vi "_OLS_Main_Rev4.vi"() -> ()   [LabVIEW 2024]
uses:
  Control Definitions/Def_PumpSpeed.ctl
  Control Definitions/Def TestState.ctl
  Control Definitions/DEF_PumpCtlRefs.ctl
  Control Definitions/DEF_Results.ctl
  Control Definitions/DEF_ Results3.ctl
  Control Definitions/Def_ATPStatus.ctl
  Control Definitions/DEF_TestInfo.ctl
  Control Definitions/Registry Keys.ctl
  Control Definitions/Global 2.vi
  Control Definitions/Global 1.vi
panel:
  out "Report Path":path
  out "Pefump VISA Ref":refnum<visa-resource-name>
  out "Test Info":T1={"Job Number"="", "Unit Number"="", "Serial Number"="", "Technician Name"="", "Calibration Date"="Cal Date", "Calibrator"="Cal by", "Calibration Slope"="M", "Calibration Offset"="B", "Config File Name"="Cal Date"}
  out "Results":T2 {"Resistor 2" format="%.1f"; "Drain" format="%.3f"; "Resistor" format="%.1f"; "Fill" format="%.3f"}
  in  "End Prog":bool=TRUE
  out "Test Index Out":i32
  out "PumpCtlRef out":T5
  out "TEST State Out":T6
  in  "Pump Speed":T7
  out "Ch B  Sim":dbl=101.0
  out "Ch A  Sim":dbl=200.0
  out "Root Path":path=path "C:/AllenProjects/PWC-OLS"
  out "Time(ms)":dbl=1249.4499999994114
  in  "ChA":dbl(slide)=24.489795918367346 scale=0.0..1200.0
  in  "ChB":dbl(slide)=36.73469387755102 scale=0.0..1200.0
  in  "ChB +100":bool
  in  "ChA +100":bool
  in  "Check":bool
  in  "DUT":i16=1
  in  "Pump JOG":bool=TRUE
  in  "Run Test":bool
  out "Pump \nStatus":bool=TRUE
  out "DataQ\nStatus":bool=TRUE
  in  "Level SP":dbl(slide)=8.0 scale=8.5..2.0
  in  "Level PV":dbl(slide)=7.715118932422306 scale=8.5..2.0
  out "Level":dbl=7.715118932422306 format="%.3f"
  in  "Drain":bool
  in  "Fill":bool
  in  "Simulate":bool
  out "TEST Name":string="OLR001--cal"
  out "DataQ Input":T8(graph)={"ChA Ohms"=100.83065830421491, "ChB Ohms"=100.0340857774357, "Laser (raw)"=1.9040000438690186}
  out "Time Stamp":timestamp=timestamp(3810639016.2712703 s since 1904-01-01)
  in  "stop":bool
  out "ChB Ohms":dbl=100.0340857774357 format="%.1f"
  out "ChA Ohms":dbl=100.79497115454612 format="%.1f"
  # "Calibration & Scaling Table\n               Tank         Key          Ref\n               Scale        Level        Measure\nEmpty\n\n\nFull"
  # "8.0      1.7752      7.844\n\n2.6      6.112        3.511"
  # "CHA             Resistance     Fill     Resistance   Drain"
  # "CHB           Resistance     Fill     Resistance   Drain"
  # "PUMP"
  # "Simulated Resistor In"
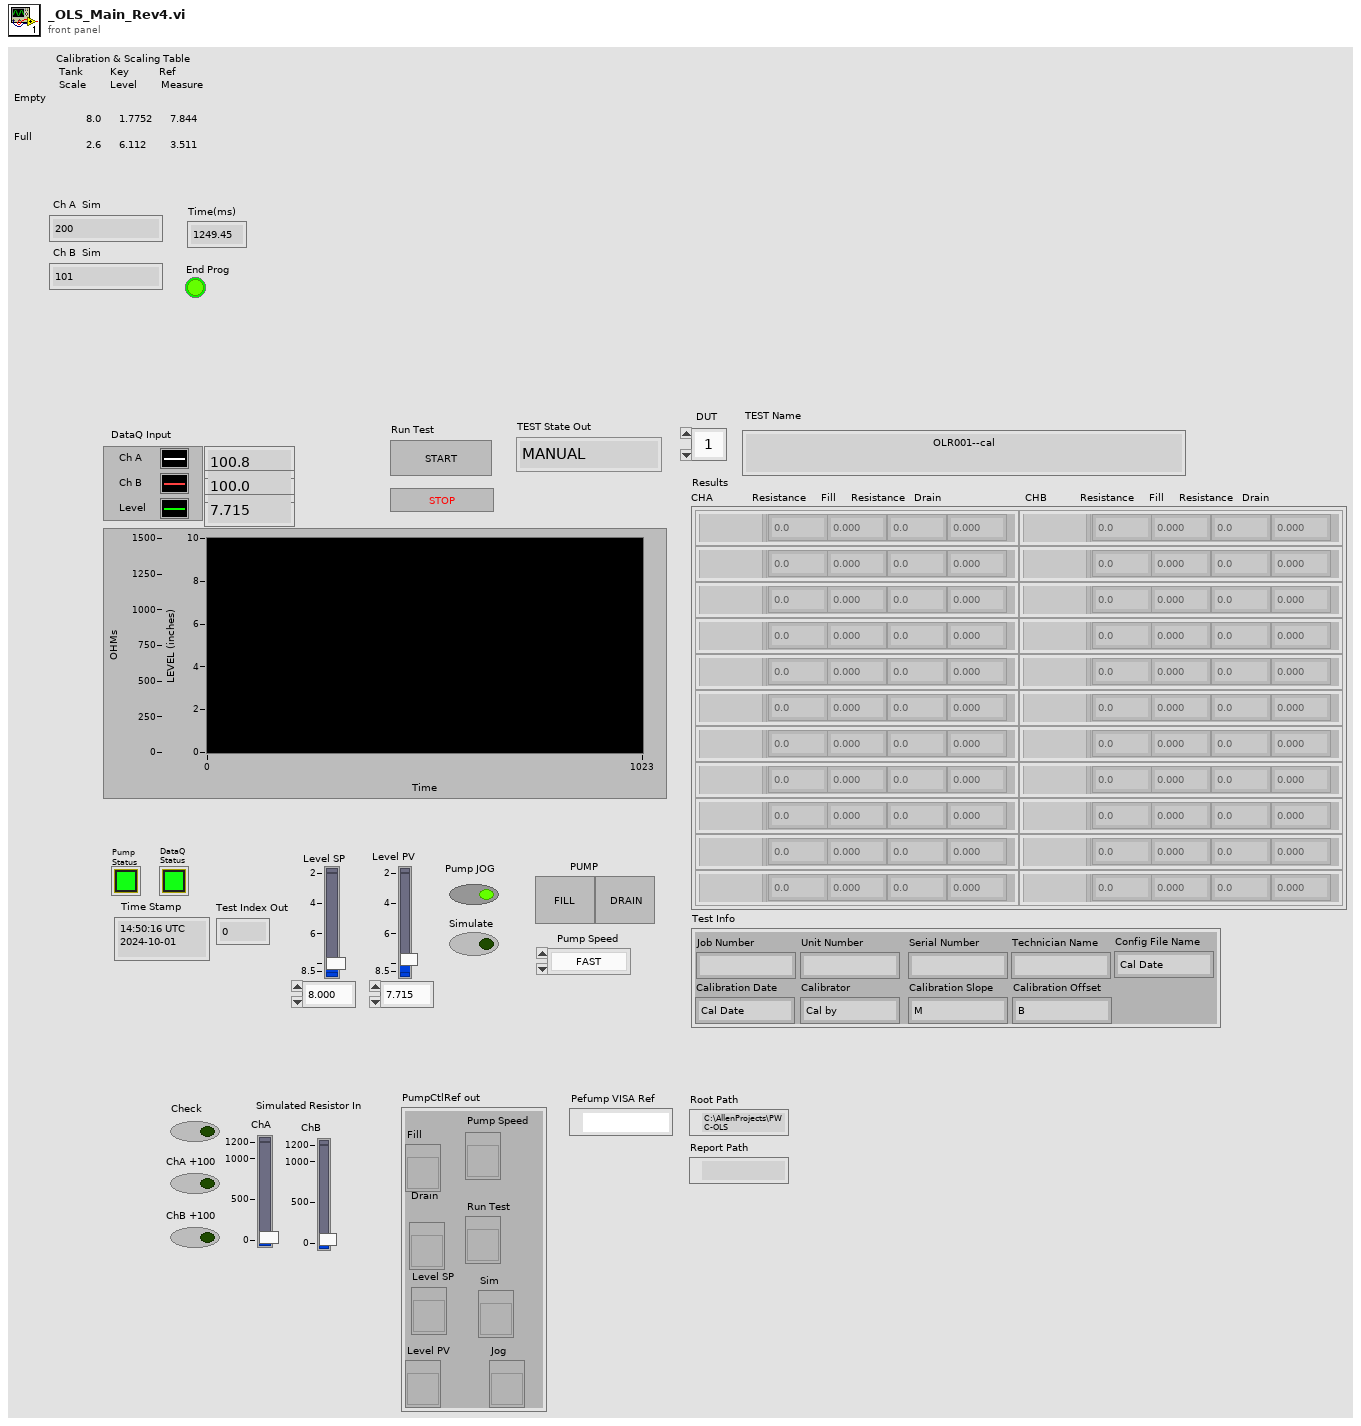
[diagram p1: front panel]
types:
  T1 = typedef "DEF_TestInfo.ctl" = cluster{"Job Number":string, "Unit Number":string, "Serial Number":string, "Technician Name":string, "Calibration Date":string, "Calibrator":string, "Calibration Slope":string, "Calibration Offset":string, "Config File Name":string}
  T2 = typedef "DEF_Results.ctl" = T3[][]
  T3 = typedef "DEF_ Results3.ctl" = cluster{"Fill":dbl, "Status":T4, "Resistor":dbl, "Drain":dbl, "Resistor 2":dbl}
  T4 = typedef "Def_ATPStatus.ctl" = i16
  T5 = typedef "DEF_PumpCtlRefs.ctl" = cluster{"Fill ":refnum<vi>, "Drain":refnum<vi>, "Level PV":refnum<vi>, "Pump Speed":refnum<vi>, "Run Test":refnum<vi>, "Sim":refnum<vi>, "Jog":refnum<vi>, "Level SP":refnum<vi>}
  T6 = typedef "Def TestState.ctl" = enum16{"MANUAL", "Start", "Pre-Fill", "Pre-Fill Measure", "Pre-Drain", "Pre-Drain Measure", "Init-Record", "Load Fill Spec", "Filling Hi", "Wait1", "Record Fill", "Load Drain Spec", "Draining Lo", "Wait2", "Record Drain", "Empty", "Done"}
  T7 = typedef "Def_PumpSpeed.ctl" = enum16{"FAST", "SLOW", "CREEP", "STOP"}
  T8 = cluster{"ChA Ohms":dbl, "ChB Ohms":dbl, "Laser (raw)":dbl}
  T9 = typedef "Registry Keys.ctl" = enum16{"Report Files Key", "Config Files Key"}
  T10 = cluster{"Pump \nStatus":refnum<vi>, "DataQ\nStatus":refnum<vi>}
  T11 = typedef "DEF_FullConfig.ctl" = cluster{"Bench Params":T12, "Test Params":dbl[][], "Pump Params":T13, "DataQ Params":T14, "Pump Control Ref":T5, "Bench Status":T15}
  T12 = typedef "DEF_BenchParams.ctl" = cluster{"Relative Root Name":string, "Values":cluster{"Step Levels":dbl, "Resistor Tolerence":dbl, "Sample Rate":dbl, "Resistor":dbl, "Wait Time":dbl}, "Report Template path":path, "Test Type":string, "Config File Name":string, "Config 2 Use":string, "Skip Pre Lube":bool}
  T13 = typedef "DEF_PumpParams.ctl" = cluster{"Empty Inches":dbl, "Full Inches":dbl, "RNG_SLOW":dbl, "RNG_CREEP":dbl, "RNG_STOP ":dbl, "VISA resource name":refnum<visa-resource-name>, "SPD_SLOW":i32, "SPD_CREEP":i32, "SPD_FAST":i32, "Zero template":path, "zero  Settle sec":i32, "Laser Slope":sgl, "Laser Offset":sgl, "Sim Fill Rate":sgl, "Cal Date":string, "Cal Technician":string}
  T14 = typedef "DEF_DataqParams.ctl" = cluster{"Visa Name":string, "Num Chan":i32, "Cal Coef":cluster{"M":dbl, "B":dbl}[], "Scale ":i32, "Cal Date":string, "Cal Technicain":string}
  T15 = typedef "DEF_BenchStatus.ctl" = cluster{"Pump Status":refnum<vi>, "Instrumnet\n Status":refnum<vi>}
  T16 = enum16{"MANUAL", "Start", "Filling", "FULL", "Draining", "EMPTY", "Done"}
  T17 = typedef "DEF_LevelOut.ctl" = cluster{"Laser ":cluster{"Raw":sgl, "Scaled":dbl}, "Level PV":dbl, "Fill":bool, "Drain":bool}
  T18 = typedef "DEF_SpecsOut.ctl" = cluster{"aSpecsTable":T19[], "Pump CtlRef In":T5, "TEST State Out":T6, "TEST Index":i32, "Drain!Fill":bool}
  T19 = typedef "Def Spec RNG.ctl" = cluster{"Specs":dbl[], "LUT Status":T20}
  T20 = typedef "Ded LUT_Status.ctl" = cluster{"ChA/!ChB":bool, "Drain/!Fill":bool, "In Range?":bool, "Switch Range?":bool, "Measure R?":bool, "Vaild R?":bool, "Index(n)":i32, "Index(n)-1":i32, "Index Max":i32, "Index(n-1)":i32}
  T21 = typedef "Def Measure.ctl" = cluster{"ChA R":dbl, "ChB R":dbl, "Level PV":dbl}
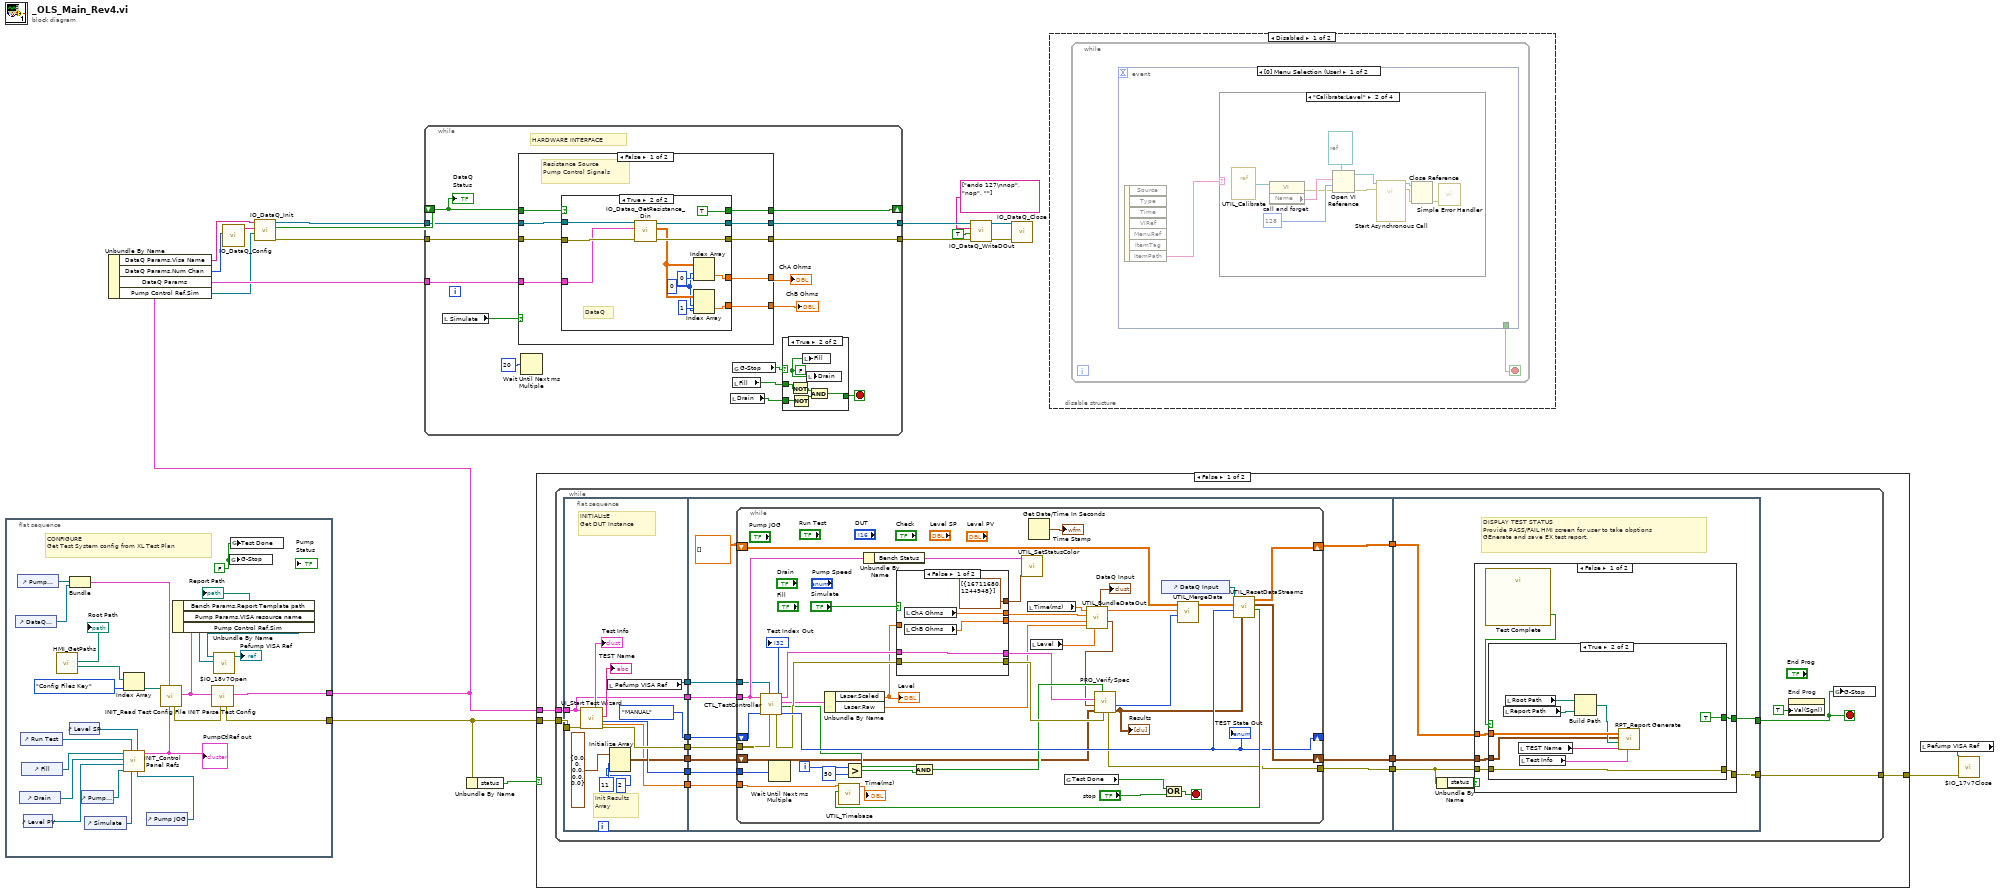
[diagram p0: block diagram]
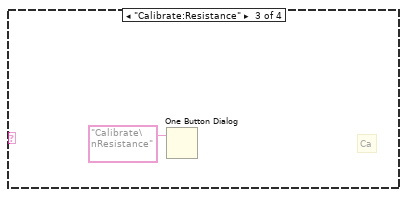
[diagram p3: hidden frame]
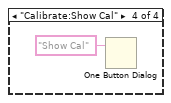
[diagram p4: hidden frame]
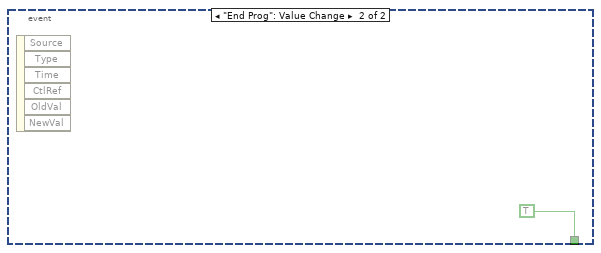
[diagram p5: hidden frame]
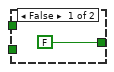
[diagram p7: hidden frame]
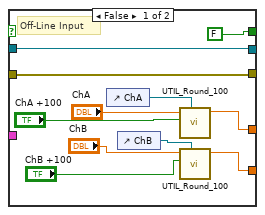
[diagram p8: hidden frame]
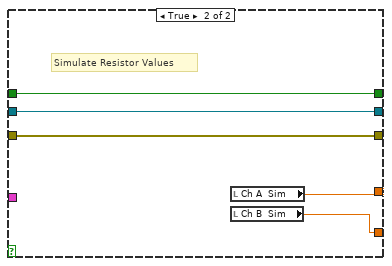
[diagram p9: hidden frame]
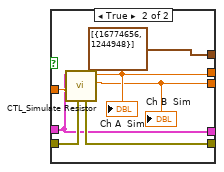
[diagram p10: hidden frame]
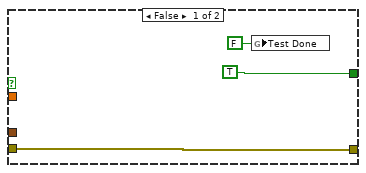
[diagram p11: hidden frame]
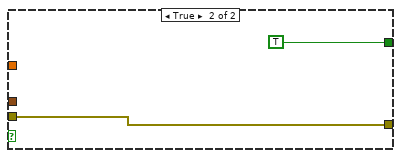
[diagram p12: hidden frame]
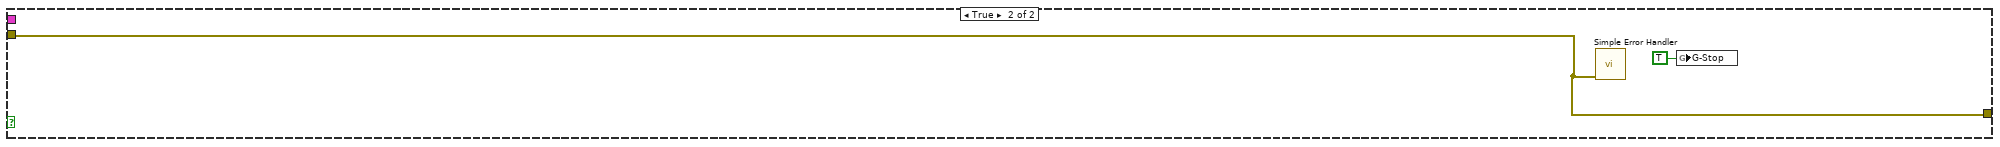
[diagram p13: hidden frame]
diagram:
  n1 = flat-sequence {
    tunnel: [w25] -> w18
    tunnel: [w39] -> w17
    frame #0 {
      w34 = FALSE ("G-Stop")
      # "CONFIGURE\nGet Test System config from XL Test Plan"
      n2 = control-ref of="DataQ\nStatus"() -> (w36:refnum<vi>)
      n3 = control-ref of="Pump \nStatus"() -> (w43:refnum<vi>)
      n4 = control-ref of="Drain"() -> (w44:refnum<vi>)
      n5 = control-ref of="Run Test"() -> (w40:refnum<vi>)
      n6 = control-ref of="Fill"() -> (w41:refnum<vi>)
      n7 = control-ref of="Level PV"() -> (w42:refnum<vi>)
      n8 = call "HMI_GetPaths.vi"() -> ("Default Paths"=w30:path[], "Root Path"=→"Root Path":path)  [unwired: 10 in]
      n9 = Bundle("Pump \nStatus"=w43, "DataQ\nStatus"=w36) -> (w28:T10)  [unwired: 1 in]
      n10 = control-ref of="Level SP"() -> (w35:refnum<vi>)
      n11 = control-ref of="Pump Speed"() -> (w32:refnum<vi>)
      n12 = control-ref of="Simulate"() -> (w38:refnum<vi>)
      n13 = Index Array(array=w30, index=Registry_Keys."Config Files Key" ("Reg Key")) -> (element=w29:path)
      n14 = control-ref of="Pump JOG"() -> (w37:refnum<vi>)
      n15 = call "INIT_Control Panel Refs.vi"("Jog"=w37, "Level SP"=w35, "Sim"=w38, "Run Test"=w40, "Pump Speed"=w32, "Level PV"=w42, "Drain"=w44, "Fill"=w41) -> ("PumpCtlRef out"=w27:T5)  [unwired: 3 in]
      "PumpCtlRef out" <- w27
      n16 = call "INIT_Read Test Config File.vi"("Pump Control Ref"=w27, "Bench Status"=w28, "Path"=w29) -> ("FullConfig"=w24:T11, "error out"=w26:errorcluster)  [unwired: 7 in]
      n17 = Unbundle By Name(w24) -> ("Bench Params.Report Template path"=→"Report Path":path, "Pump Params.VISA resource name"=w23:refnum<visa-resource-name>, "Pump Control Ref.Sim"=w20:refnum<vi>)
      n18 = call "INIT Parse Test Config.vi"("error in"=w26, "Full Config In"=w24) -> ("Full Config Out"=w39:T11, "error out"=w25:errorcluster)  [unwired: 8 in]
      n19 = call "$IO_18v7Open.vi"("Pump Control Ref.Sim"=w20, "Runtime VISA name"=w23) -> ("VISA Refnum out"=→"Pefump VISA Ref":refnum<visa-resource-name>)  [unwired: 8 in, 1 out]
      n20 = global write "Global 1.vi" "G-Stop"(w34) -> ()
      n21 = global write "Global 2.vi" "Test Done"(w34) -> ()
    }
  }
  n22 = Unbundle By Name(w17) -> ("DataQ Params.Visa Name"=w5:string, "DataQ Params.Num Chan"=w6:i32, "DataQ Params"=w4:T14, "Pump Control Ref.Sim"=w1:refnum<vi>)
  n23 = call "IO_DataQ_Config.vi"("Num Chan"=w6) -> ("Init Message"=w16:string[])  [unwired: 10 in]
  n24 = call "IO_DataQ_Init.vi"("Pump Control Ref.Sim"=w1, "Command\nList"=w16, "RunTime VISA name"=w5) -> ("error out"=w14:errorcluster, "Connected?"=w13:bool, "VISA resource name out"=w15:refnum<visa-resource-name>)  [unwired: 6 in]
  n25 = while {
    tunnel: w15 -> [w57]
    tunnel: w14 -> [w56]
    tunnel: [w54] -> w12
    tunnel: [w55] -> w10
    shift-right: [w53] -> _
    shift-left: w13 -> [w52]
    tunnel: w4 -> [w45]
    stop <- w49 stop-if-true
    # "HARDWARE INTERFACE"
    n26 = local read "Simulate"() -> (w51:bool)
    n27 = case shown="False" w51 {
      tunnel: [w75 w100] -> w58
      tunnel: [w74 w99] -> w46
      tunnel: w57 -> [w68 w102]
      tunnel: w56 -> [w69 w101]
      tunnel: [w73 w101] -> w55
      tunnel: [w72 w102] -> w54
      tunnel: [w71 w103] -> w53
      tunnel: w52 -> [w70 w103]
      tunnel: w45 -> [w67 _]
      frame False {
        # "Resistance Source\nPump Control Signals"
        n28 = case shown="True" w70 {
          tunnel: [w79 w95] -> w75
          tunnel: [w80 w92] -> w74
          tunnel: [w81 w98] -> w72
          tunnel: [w82 w97] -> w73
          tunnel: [FALSE TRUE] -> w71
          tunnel: w69 -> [w82 w88]
          tunnel: w68 -> [w81 w89]
          tunnel: w67 -> [_ w87]
          frame False {
            # "Off-Line Input"
            n29 = control-ref of="ChA"() -> (w78:refnum<vi>)
            n30 = control-ref of="ChB"() -> (w76:refnum<vi>)
            n31 = call "UTIL_Round_100.vi"("Num Refnum"=w78, "100"="ChA +100", "IN"="ChA") -> ("OUT"=w80:dbl)  [unwired: 8 in]
            n32 = call "UTIL_Round_100.vi"("Num Refnum"=w76, "100"="ChB +100", "IN"="ChB") -> ("OUT"=w79:dbl)  [unwired: 8 in]
          }
          frame True {
            w91 = 0 ("disabled index (col)")
            # "DataQ"
            n33 = call "IO_Dataq_GetResistance_Din.vi"("error in (no error)"=w88, "Dataq Params"=w87, "VISA Refnum in"=w89) -> ("error out"=w97:errorcluster, "Analog"=w93:dbl[][], "VISA Refnum out"=w98:refnum<visa-resource-name>)  [unwired: 5 in, 1 out]
            n34 = Index Array(array=w93, index (row)=0 ("index"), index (col)=w91) -> (element=w92:dbl)
            n35 = Index Array(array=w93, index (row)=w91, index (col)=1 ("index")) -> (element=w95:dbl)
          }
        }
      }
      frame True {
        # "Simulate Resistor Values"
        n36 = local read "Ch A  Sim"() -> (w99:dbl)
        n37 = local read "Ch B  Sim"() -> (w100:dbl)
      }
    }
    "ChA Ohms" <- w46
    "ChB Ohms" <- w58
    n38 = Wait Until Next ms Multiple(millisecond multiple=u32 20) -> ()  [unwired: 1 out]
    n39 = local read "Drain"() -> (w47:bool)
    n40 = local read "Fill"() -> (w48:bool)
    n41 = global read "Global 1.vi" "G-Stop"() -> (w50:bool)
    n42 = case shown="True" w50 {
      tunnel: [FALSE w62] -> w49
      tunnel: w48 -> [_ w64]
      tunnel: w47 -> [_ w61]
      frame False {
      }
      frame True {
        w66 = FALSE
        n43 = Not(x=w64) -> (.not. x?=w65:bool)
        n44 = Not(x=w61) -> (.not. x?=w63:bool)
        n45 = local write "Fill"(w66) -> ()
        n46 = local write "Drain"(w66) -> ()
        n47 = And(x=w65, y=w63) -> (x .and. y?=w62:bool)
      }
    }
    "DataQ\nStatus" <- w52
  }
  n48 = Unbundle By Name(w18) -> ("status"=w19:bool)
  n49 = case shown="False" w19 {
    tunnel: w18 -> [w106 w229]
    tunnel: [w105 w229] -> w3
    tunnel: w17 -> [w104 _]
    frame False {
      n50 = while {
        tunnel: w106 -> [w118]
        tunnel: [w112] -> w105
        tunnel: w104 -> [w108]
        stop <- w110 stop-if-true
        n51 = flat-sequence {
          tunnel: [w132] -> w120
          tunnel: [w133] -> w119
          tunnel: w118 -> [w134]
          tunnel: [w123] -> w117
          tunnel: [T16."MANUAL" ("TEST STATUS Out")] -> w116
          tunnel: [w128] -> w115
          tunnel: [w127] -> w111
          tunnel: w108 -> [w123]
          tunnel: [w122] -> w107
          tunnel: [w139] -> w121
          tunnel: w120 -> [w144]
          tunnel: w119 -> [w145]
          tunnel: w117 -> [w136]
          tunnel: w116 -> [w137]
          tunnel: w115 -> [w143]
          tunnel: [w142] -> w114
          tunnel: [w141] -> w113
          tunnel: w111 -> [w140]
          tunnel: w107 -> [w135]
          tunnel: w121 -> [w208]
          tunnel: [w207] -> w110
          tunnel: [w205] -> w112
          tunnel: w114 -> [w204]
          tunnel: w113 -> [w203]
          frame #0 {
            # "Init Results\nArray"
            # "INITIALIzE\nGet DUT Instance"
            n52 = call "UI_Start Test Wizard.vi"("error in (no error)"=w134, "Full Config"=w123) -> ("error out"=w133:errorcluster, "Time Base mS"=w132:i32, "Title"=→"TEST Name":string, "Sample Rate"=w127:dbl, "Test Info"=→"Test Info":T1)  [unwired: 3 in]
            n53 = local read "Pefump VISA Ref"() -> (w122:refnum<visa-resource-name>)
            n54 = Initialize Array(T3 {"Fill"=0.0, "Status"=0, "Resistor"=0.0, "Drain"=0.0, "Resistor 2"=0.0} ("Cluster 2"), 11 ("dimension size"), 2 ("dimension size")) -> (w128:T3[][])
          }
          frame #1 {
            n55 = while {
              tunnel: w144 -> [w188]
              tunnel: w145 -> [w179]
              tunnel: [w166] -> w139
              shift-right: [w173] -> w141
              shift-left: w143 -> [w152]
              tunnel: w140 -> [w178]
              shift-right: [w174] -> w142
              shift-left: dbl[][] [] ("Array") -> [w161]
              shift-right: [w170] -> _
              shift-left: w137 -> [w169]
              tunnel: w136 -> [w150]
              tunnel: w135 -> [w146]
              i -> [w177]
              stop <- w185 stop-if-true
              n56 = call "CTL_TestController.vi"("error in (no error)"=w179, "VISA Refnum In"=w146, "TEST State In"=w169, "FullConfig"=w150) -> ("TEST State Out"=w170:T6, "Enable"=w154:bool, "Level Out"=w149:T17, "Specs Out"=w156:T18, "error out"=w155:errorcluster, "Test Index Out"=→"Test Index Out":i32)  [unwired: 2 in]
              "TEST State Out" <- w170
              n57 = Wait Until Next ms Multiple(millisecond multiple=w188) -> ()  [unwired: 1 out]
              n58 = Unbundle By Name(w149) -> ("Laser.Scaled"=w147:dbl, "Laser.Raw"=w148:sgl)
              "Level" <- w147
              n59 = Greater?(x=w177, y=50) -> (0:w175:bool)
              n60 = Unbundle By Name(w150) -> ("Bench Status"=w186:T15)
              n61 = case shown="False" "Simulate" {
                tunnel: w155 -> [w195 w198]
                tunnel: [w195 w201] -> w168
                tunnel: [cluster{u32, u32}[] [{16711680, 1244948}] ("Normal") cluster{u32, u32}[] [{16774656, 1244948}] ("Sim Color")] -> w187
                tunnel: [w193 w200] -> w181
                tunnel: [w192 w199] -> w180
                tunnel: w156 -> [w191 w196]
                tunnel: w147 -> [_ w197]
                tunnel: [w191 w196] -> w165
                frame False {
                  n62 = local read "ChA Ohms"() -> (w193:dbl)
                  n63 = local read "ChB Ohms"() -> (w192:dbl)
                }
                frame True {
                  n64 = call "CTL_Simulate Resistor.vi"("error in (no error)"=w198, "Level IN"=w197, "Specs IN"=w196) -> ("Ch B  Ohms"=w199:dbl, "Ch A  Ohms"=w200:dbl, "error out"=w201:errorcluster)  [unwired: 6 in]
                  "Ch A  Sim" <- w200
                  "Ch B  Sim" <- w199
                }
              }
              n65 = And(x=w154, y=w175) -> (x .and. y?=w167:bool)
              n66 = call "UTIL_SetStatusColor.vi"("Colors [4] in"=w187, "Bench Status"=w186) -> ()  [unwired: 10 in]
              n67 = local read "Time(ms)"() -> (w182:dbl)
              n68 = Get Date/Time In Seconds() -> (seconds since 1Jan1904=→"Time Stamp":timestamp)
              n69 = local read "Level"() -> (w157:dbl)
              n70 = global read "Global 2.vi" "Test Done"() -> (w183:bool)
              n71 = call "UTIL_BundleDataOut.vi"("Level PV"=w157, "Laser (raw)"=w148, "ChB Ohms"=w180, "ChA Ohms"=w181, "Time (ms)"=w182) -> ("Measure"=w164:T21, "Data Out"=w163:dbl[], "Chart Data"=→"DataQ Input":T8)  [unwired: 3 in, 1 out]
              n72 = call "PRO_VerifySpec.vi"("error in (no error)"=w168, "Enable"=w167, "Results in"=w152, "Measure In"=w164, "Specs In"=w165) -> ("Results out"=w151:T2, "Status Code"=w162:i32, "error out"=w166:errorcluster)  [unwired: 4 in]
              "Results" <- w151
              n73 = control-ref of="DataQ Input"() -> (w158:refnum<vi>)
              n74 = Or(x=w183, y="stop") -> (x .or. y?=w185:bool)
              n75 = call "UTIL_MergeData.vi"("Status Code"=w162, "New Data"=w163, "Data In"=w161) -> ("Data out"=w160:dbl[][])  [unwired: 8 in]
              n76 = call "UTIL_ResetDataStreams.vi"("Results in"=w151, "TEST State Out"=w170, "Data in"=w160, "WaveformChart in"=w158) -> ("Value (Signaling)"=w171:bool, "Results out"=w173:T2, "Array"=w174:dbl[][])  [unwired: 5 in]
              n77 = call "UTIL_Timebase.vi"("Reset"=w171, "Sample Rate"=w178) -> ("Time(ms)"=→"Time(ms)":dbl)  [unwired: 9 in]
            }
          }
          frame #2 {
            # "DISPLAY TEST STATUS\nProvide PASS/FAIL HMI screen for user to take obptions\nGEnerate and save EX test report."
            n78 = Unbundle By Name(w208) -> ("status"=w206:bool)
            n79 = case shown="False" w206 {
              tunnel: w208 -> [w212 w227]
              tunnel: [w213 TRUE] -> w207
              tunnel: [w211 w227] -> w205
              tunnel: w204 -> [w210 _]
              tunnel: w203 -> [w209 _]
              frame False {
                n80 = call "Test Complete"() -> ("SAVE"=w214:bool)  [unwired: 18 in, 1 out]
                n81 = case shown="True" w214 {
                  tunnel: [TRUE TRUE] -> w213
                  tunnel: w212 -> [w216 w225]
                  tunnel: [w216 w225] -> w211
                  tunnel: w210 -> [_ w224]
                  tunnel: w209 -> [_ w219]
                  frame False {
                    n82 = global write "Global 2.vi" "Test Done"(FALSE ("Test Done")) -> ()
                  }
                  frame True {
                    n83 = local read "Report Path"() -> (w218:path)
                    n84 = local read "Root Path"() -> (w223:path)
                    n85 = local read "TEST Name"() -> (w221:string)
                    n86 = local read "Test Info"() -> (w220:T1)
                    n87 = Build Path(base path=w223, name or relative path=w218) -> (appended path=w222:path)
                    n88 = call "RPT_Report Generate.vi"("Test Info"=w220, "Report Name"=w221, "template"=w222, "Results IN"=w219, "Wave Data"=w224) -> ()  [unwired: 7 in]
                  }
                }
              }
              frame True {
              }
            }
          }
        }
        n89 = property on="End Prog" class="Bool (strict)"("Val(Sgnl)"=TRUE ("End Prog")) -> ()  [unwired: 2 in, 2 out]
        n90 = global write "Global 1.vi" "G-Stop"(w110) -> ()
      }
    }
    frame True {
      n91 = call <vilib>:"Simple Error Handler.vi"("error in (no error)"=w229) -> ()  [unwired: 4 in, 5 out]
      n92 = global write "Global 1.vi" "G-Stop"(TRUE ("G-Stop")) -> ()
    }
  }
  n93 = call "IO_DataQ_WriteDOut.vi"("error in (no error)"=w10, "Msg Active"=TRUE, "Message"=string[] ["endo 127\nnop", "nop", ""], "VISA Refnum in"=w12) -> ("error out"=w9:errorcluster, "VISA Refnum out"=w11:refnum<visa-resource-name>)  [unwired: 6 in]
  n94 = call "IO_DataQ_Close.vi"("error in"=w9, "VISA resource name"=w11) -> ()  [unwired: 10 in]
  n95 = disable-structure shown="Disabled" {
    frame Disabled {
      n96 = while {
        stop <- w231 stop-if-true
        n97 = event shown="[0] Menu Selection (User)" {
          selector: _ -> [_ _]
          dyn-events: _ -> [_ _]
          timeout: _ -> [_ _]
          tunnel: [_ TRUE] -> w231
          event Menu Selection (User) {
            n98 = event-data() -> ("ItemPath"=w232:string)  [unwired: 1 in, 6 out]
            n99 = case shown="\"Calibrate:Level\"" w232 {
              frame "False", Default {
              }
              frame "Calibrate:Level" {
                w243 = 128  # call and forget
                n100 = vi-ref "UTIL_Calibrate.vi"() -> (w236:refnum<vi>)
                n101 = property class="VI"(reference=w236) -> (error out=w234:errorcluster, "Name"=w235:string)  [unwired: 1 in, 1 out]
                n102 = Open VI Reference(type specifier VI Refnum (for type only)=refnum<vi> refnum, vi path=w235, options=w243, error in (no error)=w234) -> (vi reference=w241:refnum<vi>, error out=w240:errorcluster)  [unwired: 2 in]
                n103 = call-by-ref "Start Asynchronous Call"(reference=w241, error in=w240) -> (reference out=w238:refnum<vi>, error out=w239:errorcluster, "Digital in"=w233:refnum<vi>)  [unwired: 10 in, 1 out]
                n104 = Close Reference(reference=w238, error in (no error)=w239) -> (error out=w237:errorcluster)
                n105 = call <vilib>:"Simple Error Handler.vi"("error in (no error)"=w237) -> ()  [unwired: 4 in, 5 out]
              }
              frame "Calibrate:Resistance" {
                # "Ca"
                n106 = One Button Dialog(message="Calibrate\nResistance") -> ()  [unwired: 1 in, 1 out]
              }
              frame "Calibrate:Show Cal" {
                n107 = One Button Dialog(message="Show Cal") -> ()  [unwired: 1 in, 1 out]
              }
            }
          }
          event "End Prog": Value Change {
            n108 = event-data() -> ()  [unwired: 1 in, 6 out]
          }
        }
      }
    }
    frame Enabled {
    }
  }
  n109 = local read "Pefump VISA Ref"() -> (w2:refnum<visa-resource-name>)
  n110 = call "$IO_17v7Close.vi"("error in (no error)"=w3, "VISA Refnum in"=w2) -> ()  [unwired: 10 in]
